vi "Send Cycle Pulse.vi"(8 "error in (no error)":errorcluster, 10 "Pulse Parameter":T1, 11 "Controller in":refnum<class "Controller.lvclass">) -> (0 "error out":errorcluster, 1 "Read Voltage Setting":dbl, 2 "Read Counts:":dbl, 3 "Controller Out":refnum<class "Controller.lvclass">, 5 "Time Before OPC?":dbl)   [LabVIEW 2020, in "Controller.lvlib" / "Controller.lvclass"]
uses:
  Controller.lvclass
  Controller.lvclass/Controller.ctl
  Actor_AFG/Actor_AFG Messages/Setup Pulse Waveform Msg/Setup Pulse Waveform Msg.lvclass/Setup Pulse Waveform Msg.ctl
  <vilib>/ActorFramework/Message Enqueuer/Message Enqueuer.lvclass/Message Enqueuer.ctl
  Actor_AFG/Actor_AFG Messages/AFG Setup Cycle Msg/AFG Setup Cycle Msg.lvclass/AFG Setup Cycle Msg.ctl
  Actor_AFG/Actor_AFG Messages/AFG Enable Output Msg/AFG Enable Output Msg.lvclass/AFG Enable Output Msg.ctl
  <vilib>/ActorFramework/Message Enqueuer/Enqueue.vi
  Actor_AFG/Actor_AFG Messages/Setup Pulse Waveform Msg/Setup Pulse Waveform Msg.lvclass
  C:/Program Files/National Instruments/LabVIEW 2020/vi.lib/ActorFramework/Message/Message.lvclass
  Actor_AFG/Actor_AFG Messages/AFG Setup Cycle Msg/AFG Setup Cycle Msg.lvclass
  Actor_AFG/Actor_AFG Messages/AFG Enable Output Msg/AFG Enable Output Msg.lvclass
  Actor_NI6008/Actor_NI6008 Messages/NI6008 Enout Trigger Msg/NI6008 Enout Trigger Msg.lvclass
  <vilib>/ActorFramework/Message Priority Queue/Priority Enqueue.vi
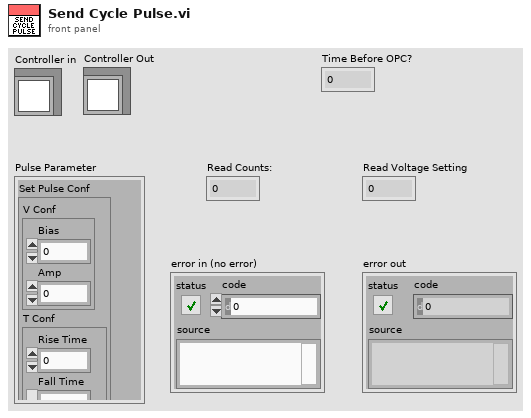
[diagram p1: front panel]
types:
  T1 = cluster{"Set Pulse Conf":cluster{"V Conf":cluster{"Bias":dbl, "Amp":dbl}, "T Conf":cluster{"Rise Time":dbl, "Fall Time":dbl, "Pulse Width":dbl}}, "Reset Pulse Conf":cluster{"V Conf":cluster{"Bias":dbl, "Amp":dbl}, "T Conf":cluster{"Rise Time":dbl, "Fall Time":dbl, "Pulse Width":dbl}}, "Cycle Timing":cluster{"Delay":dbl, "Pulse Spacing":dbl, "Burst Counts:":dbl, "Read Counts:":dbl}, "Read Voltage Setting":dbl}
  T2 = cluster{"V Conf":cluster{"Bias":dbl, "Amp":dbl}, "T Conf":cluster{"Rise Time":dbl, "Fall Time":dbl, "Pulse Width":dbl}}
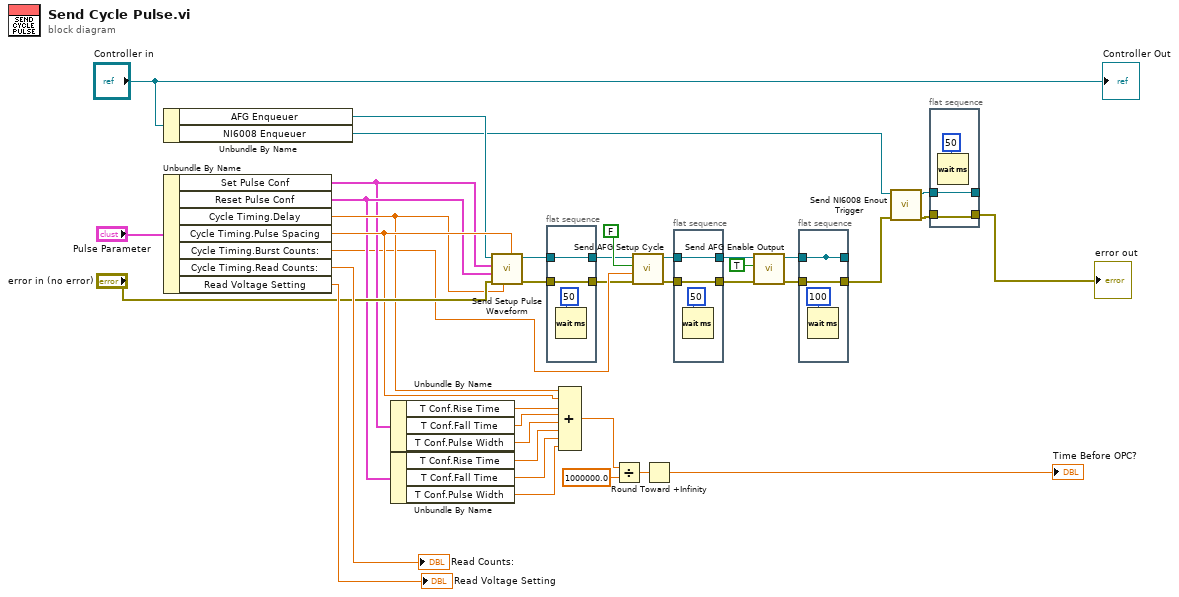
[diagram p0: block diagram]
diagram:
  n1 = Unbundle By Name("Controller in") -> ("AFG Enqueuer"=w5:refnum<class "Message Enqueuer.lvclass">, "NI6008 Enqueuer"=w3:refnum<class "Message Enqueuer.lvclass">)
  n2 = Unbundle By Name("Pulse Parameter") -> ("Set Pulse Conf"=w17:T2, "Reset Pulse Conf"=w18:T2, "Cycle Timing.Delay"=w25:dbl, "Cycle Timing.Pulse Spacing"=w26:dbl, "Cycle Timing.Burst Counts:"=w13:dbl, "Cycle Timing.Read Counts:"=→"Read Counts:":dbl, "Read Voltage Setting"=→"Read Voltage Setting":dbl)
  n3 = Unbundle By Name(w17) -> ("T Conf.Rise Time"=w19:dbl, "T Conf.Fall Time"=w20:dbl, "T Conf.Pulse Width"=w21:dbl)
  n4 = Unbundle By Name(w18) -> ("T Conf.Rise Time"=w22:dbl, "T Conf.Fall Time"=w23:dbl, "T Conf.Pulse Width"=w24:dbl)
  n5 = call "Send Setup Pulse Waveform.vi"("Spacing"=w26, "Delay"=w25, "error in (no error)"="error in (no error)", "Reset Pulse Conf"=w18, "Set Pulse Conf"=w17, "Message Enqueuer"=w5) -> ("error out"=w12:errorcluster, "Message Enqueuer out"=w11:refnum<class "Message Enqueuer.lvclass">)  [unwired: 4 in]
  n6 = flat-sequence {
    tunnel: w11 -> [w41]
    tunnel: [w41] -> w6
    tunnel: [w40] -> w7
    tunnel: w12 -> [w40]
    frame #0 {
      n7 = Wait (ms)(milliseconds to wait=u32 50) -> ()  [unwired: 1 out]
    }
  }
  n8 = Compound Arithmetic op=ADD(w25, w26, w19, w20, w21, w22, w23, w24) -> (w28:dbl)
  n9 = Divide(x=w28, y=1000000.0) -> (x/y=w29:dbl)
  n10 = call "Send AFG Setup Cycle.vi"("error in (no error)"=w7, "Cycles"=w13, "Continuous"=FALSE ("Repeat"), "Message Enqueuer"=w6) -> ("error out"=w10:errorcluster, "Message Enqueuer out"=w9:refnum<class "Message Enqueuer.lvclass">)  [unwired: 6 in]
  n11 = Round Toward +Infinity(x=w29) -> (ceil(x): smallest int >= x=→"Time Before OPC?":dbl)
  n12 = flat-sequence {
    tunnel: w9 -> [w43]
    tunnel: w10 -> [w42]
    tunnel: [w43] -> w34
    tunnel: [w42] -> w35
    frame #0 {
      n13 = Wait (ms)(milliseconds to wait=u32 50) -> ()  [unwired: 1 out]
    }
  }
  n14 = call "Send AFG Enable Output.vi"("error in (no error)"=w35, "Enable Output (T: Enable)"=TRUE, "Message Enqueuer"=w34) -> ("error out"=w36:errorcluster, "Message Enqueuer out"=w37:refnum<class "Message Enqueuer.lvclass">)  [unwired: 7 in]
  n15 = flat-sequence {
    tunnel: [w45] -> _
    tunnel: w36 -> [w46]
    tunnel: [w45] -> _
    tunnel: [w46] -> w2
    tunnel: w37 -> [w45]
    frame #0 {
      n16 = Wait (ms)(milliseconds to wait=u32 100) -> ()  [unwired: 1 out]
    }
  }
  n17 = call "Send NI6008 Enout Trigger.vi"("error in (no error)"=w2, "Message Enqueuer"=w3) -> ("error out"=w16:errorcluster, "Message Enqueuer out"=w15:refnum<class "Message Enqueuer.lvclass">)  [unwired: 8 in]
  n18 = flat-sequence {
    tunnel: w15 -> [w49]
    tunnel: w16 -> [w48]
    tunnel: [w49] -> _
    tunnel: [w48] -> w1
    frame #0 {
      n19 = Wait (ms)(milliseconds to wait=u32 50) -> ()  [unwired: 1 out]
    }
  }
  "error out" <- w1
  "Controller Out" <- "Controller in"
